vi "String builder freq range (SubVI).vi"(10 "lower":dbl, 11 "upper":dbl) -> (3 "String":string)   [LabVIEW 2017]
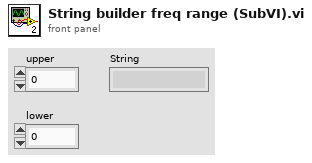
[diagram p1: front panel]
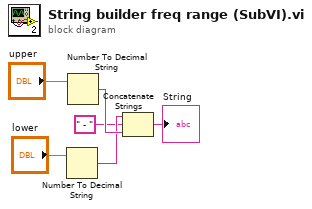
[diagram p0: block diagram]
diagram:
  n1 = Number To Decimal String(number="lower") -> (decimal integer string=w4:string)  [unwired: 1 in]
  n2 = Number To Decimal String(number="upper") -> (decimal integer string=w5:string)  [unwired: 1 in]
  n3 = Concatenate Strings(w4, " - ", w5) -> (→"String":string)
